vi "RGB2HSV.vi"(3 "B":u8, 4 "G":u8, 5 "R":u8) -> (0 "V":dbl, 1 "S":dbl, 2 "H":dbl)   [LabVIEW 2020]
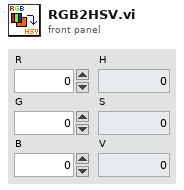
[diagram p1: front panel]
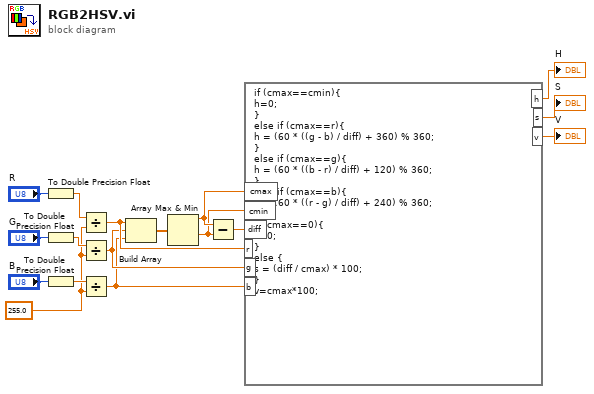
[diagram p0: block diagram]
diagram:
  w7 = 255.0 ("y")
  n1 = To Double Precision Float(number="R") -> (double precision float=w13:dbl)
  n2 = To Double Precision Float(number="G") -> (double precision float=w12:dbl)
  n3 = To Double Precision Float(number="B") -> (double precision float=w11:dbl)
  n4 = Divide(x=w13, y=w7) -> (x/y=w10:dbl)
  n5 = Divide(x=w12, y=w7) -> (x/y=w9:dbl)
  n6 = Divide(x=w11, y=w7) -> (x/y=w8:dbl)
  n7 = Build Array(w10, w9, w8) -> (w17:dbl[])
  n8 = Array Max & Min(array=w17) -> (max value=w16:dbl, min value=w15:dbl)  [unwired: 2 out]
  n9 = Subtract(x=w16, y=w15) -> (x-y=w14:dbl)
  n10 = formula code="if (cmax==cmin){\nh=0;\n}\nelse if (cmax==r){\nh = (60 * ((g - b) / diff) + 360) % 360;\n}\nelse if (cmax==g){\nh = (60 * ((b - r) / diff) + 120) % 360;\n}\nelse if (cmax==b){\nh = (60 * ((r - g) / diff) + 240) % 360;\n}\nif (cmax==0){\ns=0;\n}\nelse {\ns = (diff / cmax) * 100;\n}\nv=cmax*100;"("cmax"=w16, "cmin"=w15, "diff"=w14, "r"=w10, "g"=w9, "b"=w8) -> ("h"=→"H":dbl, "s"=→"S":dbl, "v"=→"V":dbl)
